vi "CSConnect.UpdateOneVoltage.vi"(0 "i ref in":refnum<vi>, 2 "In-channel number":i32, 3 "In-Voltage":dbl, 5 "error in (no error)":errorcluster) -> (14 "i ref out":refnum<vi>, 19 "error out":errorcluster)   [LabVIEW 2014, in "CSConnect.lvlib"]
doc: "Updates the voltage of a channel.\n\nLicense Agreement for this software:\n\nCopyright (C)\nGesellschaft für Schwerionenforschung, GSI\nPlanckstr. 1\n64291 Darmstadt\nGermany\n\nContact: D.Beck@gsi.de \n\nThis program is free software; you can redistribute it and/or modify it under the terms of the \nGNU General Public License as published by the Free Software Foundation; either version 2 of \nthe license, or (at your option) any later version.\n\nThis program is distributed in the hope that it will be useful, but WITHOUT ANY WARRANTY; \nwithout even the implied warranty of MERCHANTABILITY or FITNESS FOR A PARTICULAR PURPOSE. See the GNU General License for more details (http://www.gnu.org).\n\nGesellschaft für Schwerionenforschung, GSI\nPlanckstr. 1, 64291 Darmstadt, Germany\nFor all questions and ideas contact: M.Richter@gsi.de, H.Brand@gsi.de or D.Beck@gsi.de.\nLast update: 16-JUN-2004"
uses:
  CSConnect.lvlib
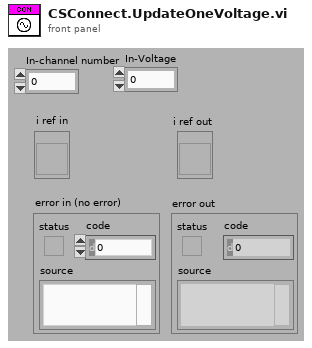
[diagram p1: front panel]
types:
  T1 = typedef "CSConnect.lvlib/CSConnect.i attribute.ctl" = cluster{"In-Array":cluster{"Alias":string, "Value":dbl, "neededOuts":bool[]}[], "Out-Array":cluster{"ObjectName":string, "VoltFunctionName":string, "OnOffFunctionName":string, "Channel":string, "Calculation-Formula":string}[], "OutChannelsID":i32, "InOutMatrixID":i32}
  T2 = cluster{"Alias":string, "Value":dbl, "neededOuts":bool[]}[]
  T3 = cluster{"Alias":string, "Value":dbl, "neededOuts":bool[]}
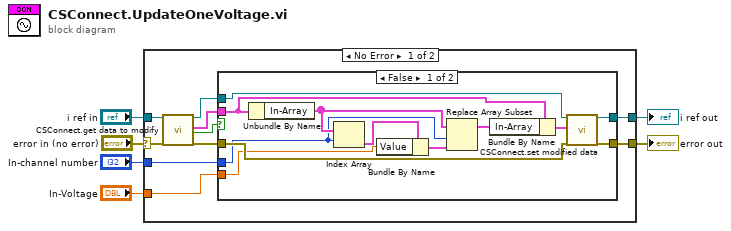
[diagram p0: block diagram]
diagram:
  n1 = case shown="No Error" "error in (no error)" {
    selector: "error in (no error)" -> [w13 w31]
    tunnel: [w10 w31] -> w6
    tunnel: [w11 w32] -> w4
    tunnel: "i ref in" -> [w14 w32]
    tunnel: "In-channel number" -> [w15 _]
    tunnel: "In-Voltage" -> [w7 _]
    frame No Error {
      n2 = call "CSConnect.get data to modify.vi"("i ref in"=w14, "error in (no error)"=w13) -> ("i ref out"=w12:refnum<vi>, "i attribute"=w16:T1, "timed out"=w8:bool, "error out"=w9:errorcluster)  [unwired: 14 in]
      n3 = case shown="False" w8 {
        tunnel: w16 -> [w28 _]
        tunnel: w15 -> [w20 _]
        tunnel: w12 -> [w25 w30]
        tunnel: [w24 w30] -> w11
        tunnel: [w23 w29] -> w10
        tunnel: w9 -> [w22 w29]
        tunnel: w7 -> [w17 _]
        frame False {
          n4 = Unbundle By Name(w28) -> ("In-Array"=w21:T2)
          n5 = Index Array(array=w21, index=w20) -> (element=w19:T3)
          n6 = Bundle By Name(cluster=w19, "Value"=w17) -> (w18:T3)
          n7 = Replace Array Subset(array=w21, new element=w18, index=w20) -> (w27:T2)
          n8 = Bundle By Name(cluster=w28, "In-Array"=w27) -> (w26:T1)
          n9 = call "CSConnect.set modified data.vi"("i ref in"=w25, "i attribute"=w26, "error in (no error)"=w22) -> ("i ref out"=w24:refnum<vi>, "error out"=w23:errorcluster)  [unwired: 15 in]
        }
        frame True {
        }
      }
    }
    frame Error {
    }
  }
  "error out" <- w6
  "i ref out" <- w4
